vi "GSP_Manager_Slit.vi"() -> ()   [LabVIEW 2015]
uses:
  SystemUtil/ScriptArray.ctl
  SystemUtil/Script.ctl
  SystemUtil/MotorStates.ctl
  SystemUtil/ThreadStates.ctl
  Log/LogItem.ctl
  GSP_SLIT_Global.vi
  GUI/GSP_GUI_global.vi
  <vilib>/Utility/file.llb/Read From Spreadsheet File (DBL).vi
panel:
  in  "SLICER IN":bool
  in  "Slit":picture caption="Mask Is Out"
  in  "Mask bump":i32(slide) scale=-30.0..30.0
  in  "Hide Slit":bool
  in  "Slit Mask#":i32(ring) items=["<NO MASK>"]
  out "Last Error":errorcluster
  in  "CommandQ":string
  # "Mask"
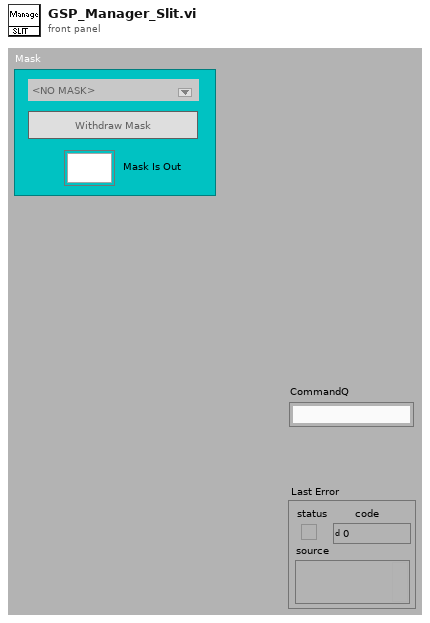
[diagram p1: front panel]
types:
  T1 = typedef "ScriptArray.ctl" = T2[]
  T2 = typedef "Script.ctl" = cluster{"Current Step":i32, "Commands":cluster{"Command":string, "Parameters":string}[]}
  T3 = cluster{"Trans Grab Mem Address":i32, "Trans Release Mem Address":i32, "Trans Home Mem Address":i32, "Trans Move Mem Address":i32, "Trans Open Mask Address":i32, "Trans Close Mask Address":i32, "Rot Home Mem Address":i32, "Rot Rotate Mem Address":i32}
  T4 = typedef "MotorStates.ctl" = enum16{"Ready", "Moving", "Uninitialized", "Error"}
  T5 = enum16{"POL (0)", "CPL (1)", "HLT (2)", "STP (3)", "RST (4)", "RVN (5)", "RPB (6)", "CLP (8)", "SDL (9)", "RUN (10)", "WRI (11)", "RRG (12)", "SPR (13)", "LPR (14)", "VMI (15)", "SSP (17)", "SSE (18)", "RIS (20)", "RIO (21)", "IMW (25)", "END (128)", "MAV (134)", "MRV (135)", "JRE (137)", "WCL (138)", "WCW (139)", "DLY (140)", "WDL (141)", "GCL (142)", "GOP (143)", "ZTG (144)", "ZTP (145)", "TTP (146)", "CME (147)", "CTC (148)", "TQL (149)", "AHC (150)", "ERL (151)", "OLP (152)", "WRP (154)", "IDT (155)", "LRP (156)", "VMP (159)", "RAV (160)", "RRV (161)", "JMP (162)", "JOI (162)", "CIS (163)", "CKS (164)", "CLC (165)", "KMC (167)", "MCT (168)", "FLC (169)", "EEM (170)", "DDB (171)", "DEM (171)", "PAC (172)", "ADL (173)", "BRT (174)", "MAT (176)", "MRT (177)", "RAT (178)", "RRT (179)", "SSD (180)", "KMR (181)", "KED (182)", "KDD (183)", "DIR (184)", "PRO (185)", "SIF (186)", "EDL (187)", "CIO (188)", "MDS (189)", "MDC (190)", "MDT (191)", "SEE (192)", "ARI (193)", "WBS (194)", "SCF (195)", "RSM (196)", "RLM (197)", "RSN (198)", "RLN (199)", "PCL (201)", "PCI (201)", "PRT (202)", "PRI (202)", "WBE (204)", "SOB (205)", "COB (206)", "ACR (207)", "PLR (208)", "CAI (211)", "LVT (212)", "OVT (213)", "MTT (214)", "CLC (215)", "PIM (216)", "VIM (217)", "TIM (218)", "AHM (219)", "SSL (221)", "TRU (222)", "RSD (223)", "EMT (225)", "DMT (226)", "EMD (227)", "DMD (228)", "HSM (229)", "AHD (230)", "PCM (231)", "PCG (232)", "XRV (233)", "XAV (234)", "XRT (235)", "XAT (236)", "GOC (237)", "JNA (238)", "JOR (239)", "PMC (240)", "PMV (241)", "PMX (242)", "DLC (243)", "SLC (244)", "PCP (245)", "ATR (248)", "PMO (249)", "JAN (250)", "EDH (251)", "DIF (252)", "IMS (253)", "IMQ (254)"}
  T6 = typedef "ThreadStates.ctl" = enum16{"Waiting", "Scripting", "Uninitialized", "Error"}
  T7 = cluster{"left":i16, "top":i16, "right":i16, "bottom":i16}
  T8 = cluster{"Width":u16, "Style":enum32{"Solid", "Dash", "Dot", "DashDot", "DashDotDot"}}
  T9 = enum16{"Launch", "Log", "Open", "Close", "Shutdown"}
  T10 = typedef "LogItem.ctl" = cluster{"error in (no error)":errorcluster, "Source":string, "Comment ":string}
  T11 = cluster{"left":i16, "bottom":i16, i16, "bottom":i16}
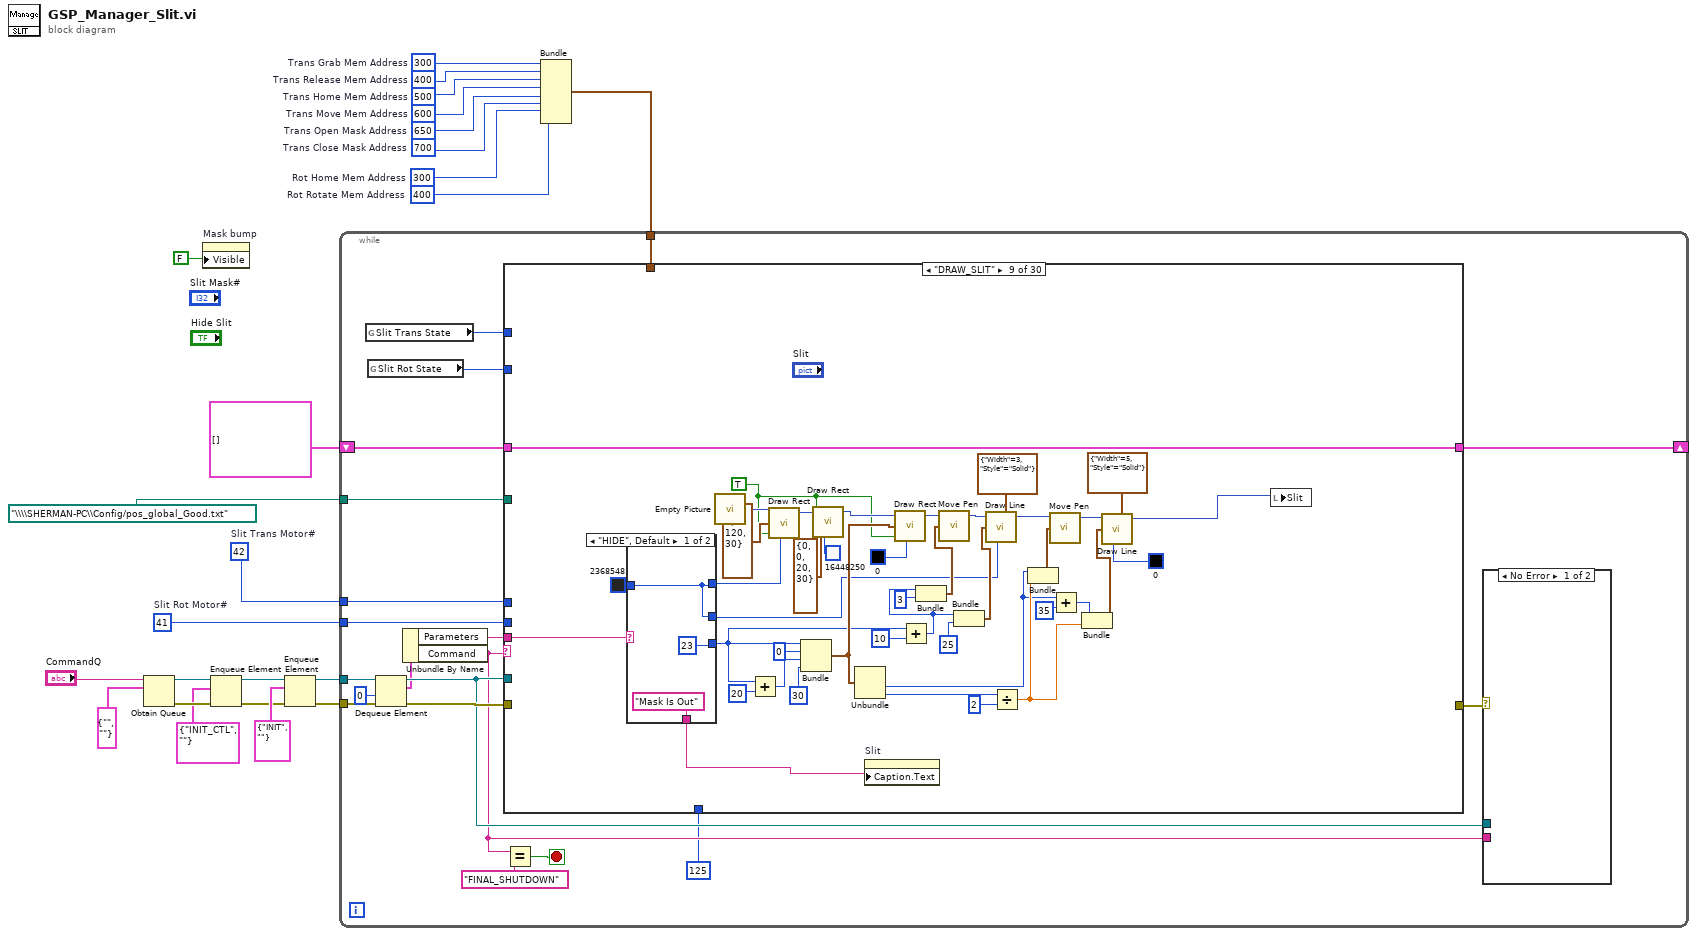
[diagram p0: block diagram]
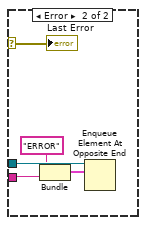
[diagram p2: hidden frame]
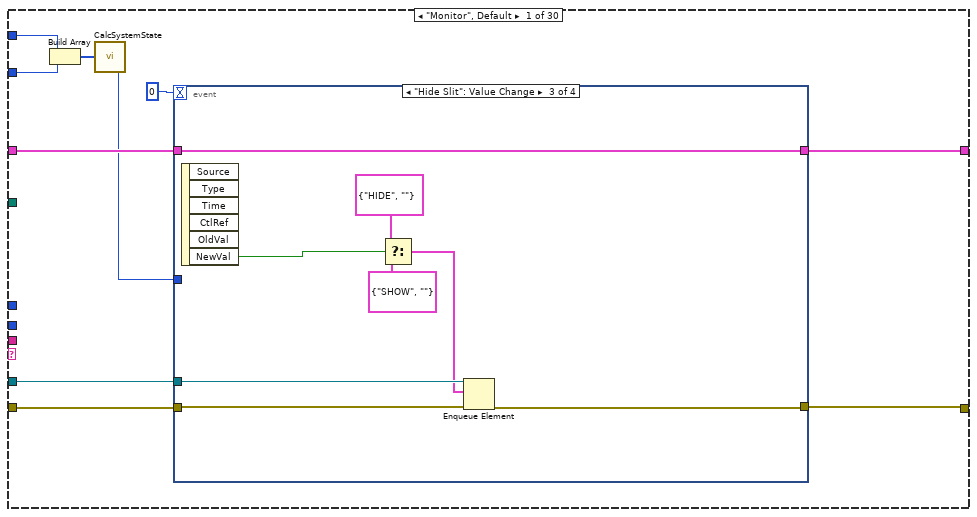
[diagram p3: hidden frame]
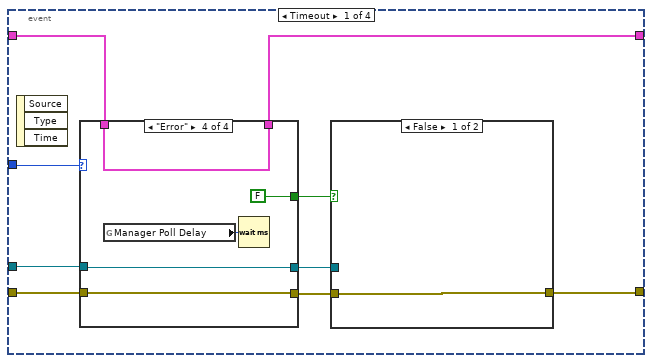
[diagram p4: hidden frame]
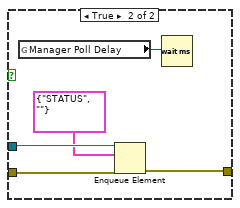
[diagram p5: hidden frame]
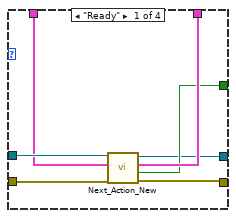
[diagram p6: hidden frame]
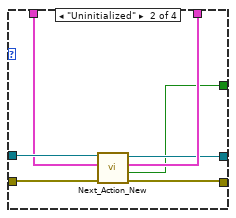
[diagram p7: hidden frame]
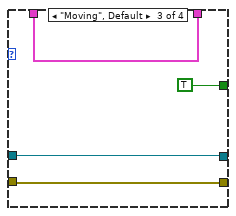
[diagram p8: hidden frame]
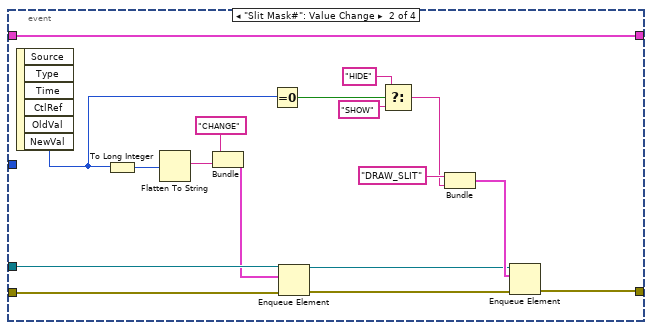
[diagram p9: hidden frame]
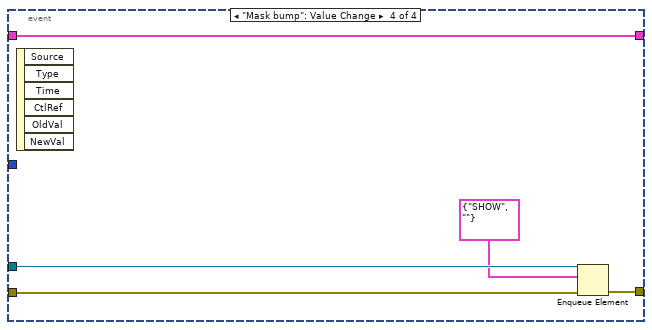
[diagram p10: hidden frame]
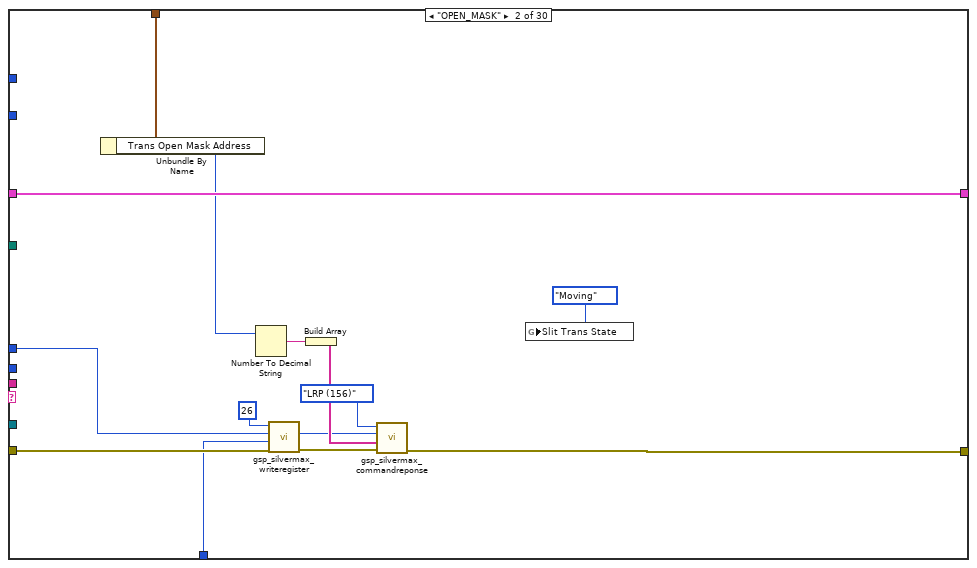
[diagram p11: hidden frame]
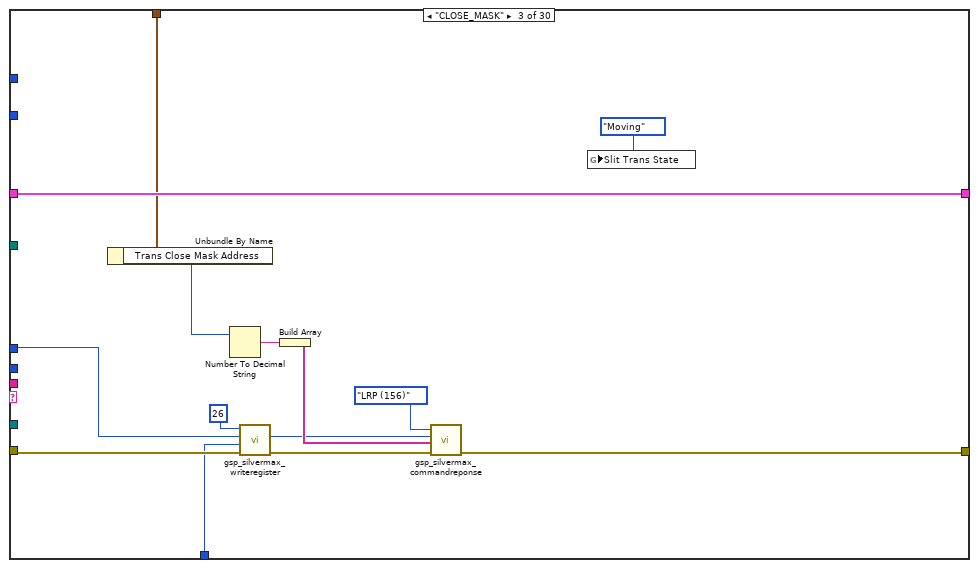
[diagram p12: hidden frame]
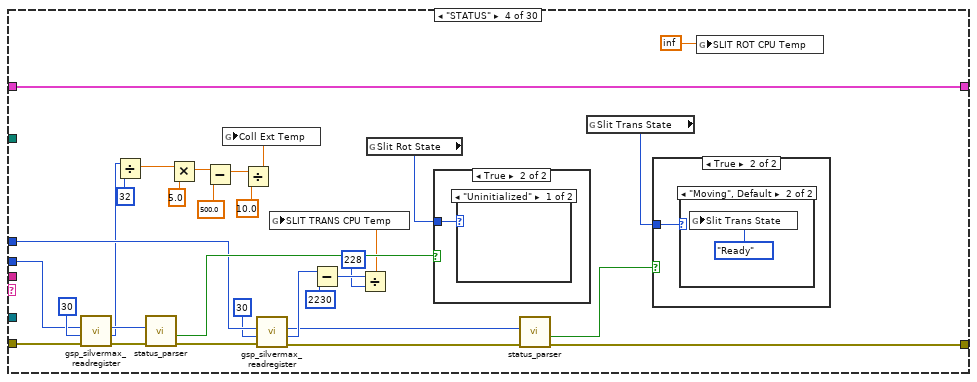
[diagram p13: hidden frame]
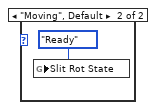
[diagram p17: hidden frame]
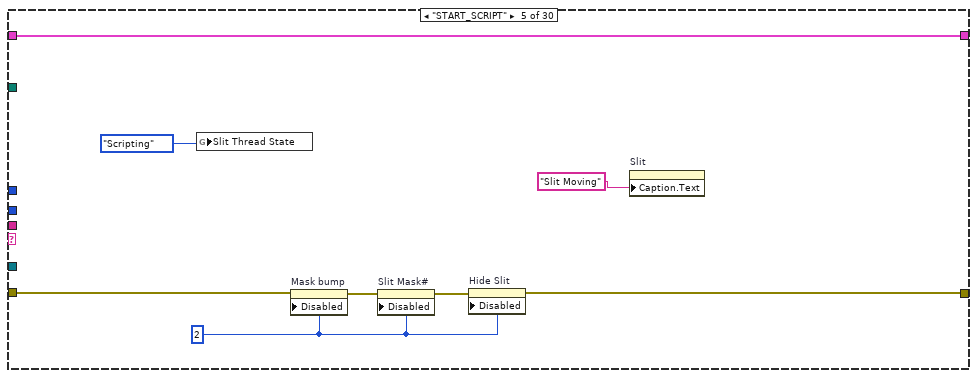
[diagram p18: hidden frame]
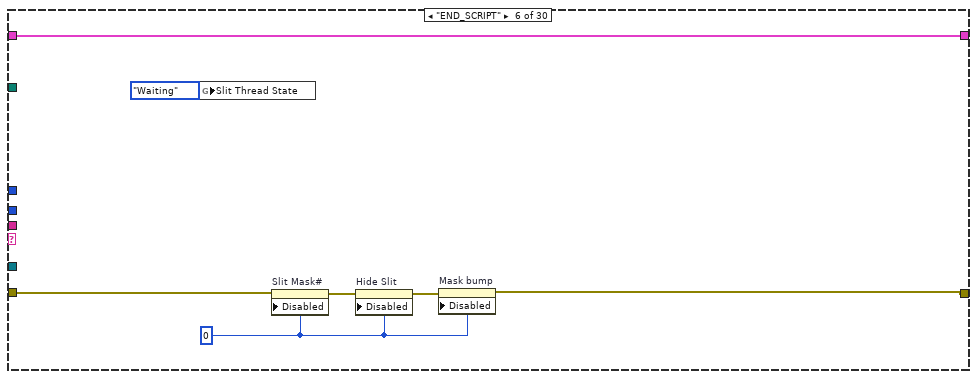
[diagram p19: hidden frame]
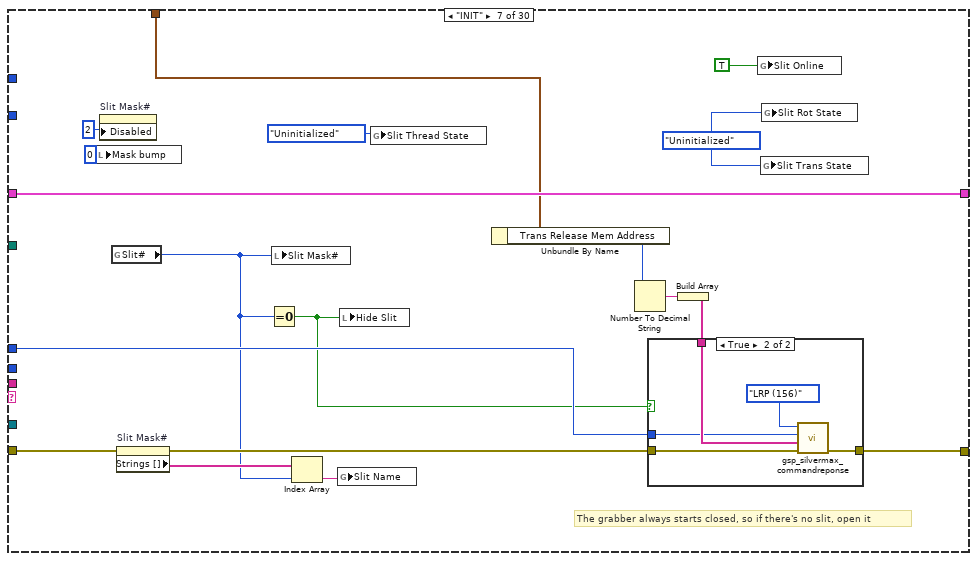
[diagram p20: hidden frame]
diagram:
  w16 = 300  # Trans Grab Mem Address
  w15 = 400  # Trans Release Mem Address
  w14 = 500  # Trans Home Mem Address
  w13 = 600  # Trans Move Mem Address
  w11 = 700  # Trans Close Mask Address
  w12 = 650  # Trans Open Mask Address
  w10 = 300  # Rot Home Mem Address
  w9 = 400  # Rot Rotate Mem Address
  w17 = u8 41  # Slit Rot Motor#
  w18 = u8 42  # Slit Trans Motor#
  n1 = Obtain Queue(name (unnamed)="CommandQ", element data type=cluster{"Command":string, "Parameters":string} {"Command"="", "Parameters"=""} ("Default Command")) -> (queue out=w4:refnum<queue>, error out=w5:errorcluster)  [unwired: 3 in, 1 out]
  n2 = property on="Mask bump" class="Slide (strict)"("Visible"=FALSE) -> ()  [unwired: 2 in, 2 out]
  n3 = Enqueue Element(queue=w4, element=cluster{"Command":string, "Parameters":string} {"Command"="INIT_CTL", "Parameters"=""}, error in (no error)=w5) -> (queue out=w7:refnum<queue>, error out=w6:errorcluster)  [unwired: 1 in, 1 out]
  n4 = Enqueue Element(queue=w7, element=cluster{"Command":string, "Parameters":string} {"Command"="INIT", "Parameters"=""}, error in (no error)=w6) -> (queue out=w24:refnum<queue>, error out=w23:errorcluster)  [unwired: 1 in, 1 out]
  n5 = Bundle("Trans Grab Mem Address"=w16, "Trans Release Mem Address"=w15, "Trans Home Mem Address"=w14, "Trans Move Mem Address"=w13, "Trans Open Mask Address"=w12, "Trans Close Mask Address"=w11, "Rot Home Mem Address"=w10, "Rot Rotate Mem Address"=w9) -> (w8:T3)  [unwired: 1 in]
  n6 = while {
    tunnel: w24 -> [w44]
    tunnel: w23 -> [w43]
    tunnel: w18 -> [w38]
    tunnel: w17 -> [w37]
    shift-right: [w36] -> _
    shift-left: T1 [] ("Operations") -> [w26]
    tunnel: w8 -> [w27]
    tunnel: path "\\\\SHERMAN-PC\\Config/pos_global_Good.txt" -> [w25]
    stop <- w33 stop-if-true
    n7 = global read "GSP_SLIT_Global.vi" "Slit Trans State"() -> (w28:T4)
    n8 = global read "GSP_SLIT_Global.vi" "Slit Rot State"() -> (w29:T4)
    n9 = Dequeue Element(queue=w44, timeout in ms (-1)=0, error in (no error)=w43) -> (queue out=w40:refnum<queue>, element=w35:cluster{"Command":string, "Parameters":string}, error out=w42:errorcluster)  [unwired: 1 out]
    n10 = Unbundle By Name(w35) -> ("Parameters"=w34:string, "Command"=w32:string)
    n11 = case shown="\"DRAW_SLIT\"" w32 {
      tunnel: w42 -> [w59 w136 w148 w182 w197 w204 w210 w239 _ w300 w310 w334 w363 w392 w397 w410 w424 w441 w459 w473 w492 w519 w545 w549 w568 w584 w626 w635 w638 _]
      tunnel: w40 -> [w50 _ _ _ _ _ _ _ _ w294 _ _ _ _ _ _ _ _ _ _ _ _ _ _ _ w590 w627 _ _ w664]
      tunnel: [w51 w128 w151 w167 w193 w201 w214 w239 _ w296 w309 w333 w365 w392 w397 w414 w419 w434 w463 w481 w494 w526 w545 w549 w577 w589 w622 w635 w650 _] -> w41
      tunnel: w38 -> [_ w135 w147 w170 _ _ w213 _ _ w298 _ _ _ _ _ w409 w423 w438 w458 w472 w493 w517 _ _ _ _ _ _ w642 _]
      tunnel: w37 -> [_ _ _ w181 _ _ _ _ _ w297 _ _ _ _ _ _ _ _ _ _ _ _ _ _ w581 _ _ _ w653 _]
      tunnel: w26 -> [w58 w141 w155 w184 w198 w205 w222 w240 w286 w301 w314 w338 w368 w396 w401 w404 w432 w439 w454 w470 w488 w522 w544 w548 w571 w592 w628 w637 w643 w658]
      tunnel: [w52 w141 w155 w184 w198 w205 w222 w240 w286 w301 w313 w337 w367 w395 w400 w404 w432 w439 w454 w470 w488 w522 w544 w548 w571 w591 w628 w636 w643 w657] -> w36
      tunnel: w34 -> [_ _ _ _ _ _ _ _ w247 _ w312 w336 w361 _ _ _ _ _ _ _ _ _ _ _ w566 _ _ _ _ _]
      tunnel: 125 ("Register Value") -> [_ w132 w145 _ _ _ _ _ _ _ _ _ _ _ _ _ _ _ _ _ _ _ _ _ _ _ _ _ _ _]
      tunnel: w29 -> [w55 _ _ _ _ _ _ _ _ _ w308 w332 _ _ _ _ _ _ _ _ _ _ _ _ _ w587 _ _ _ _]
      tunnel: w28 -> [w56 _ _ _ _ _ _ _ _ _ w307 w331 _ _ _ _ _ _ _ _ _ _ _ _ _ w588 _ _ _ _]
      tunnel: w27 -> [_ w131 w144 _ _ _ w215 _ _ _ _ _ _ _ _ w403 w422 w440 w453 w469 w487 w521 _ _ w565 _ _ _ w641 _]
      tunnel: w25 -> [_ _ _ _ _ _ _ w235 _ _ _ _ _ _ _ _ _ _ _ _ w485 w516 _ _ w555 _ _ _ _ _]
      frame "Monitor", Default {
        n12 = Build Array(w56, w55) -> (w57:T4[])
        n13 = call "CalcSystemState.vi"("Motor States"=w57) -> ("system state"=w53:T4)
        n14 = event shown="[2] \"Hide Slit\": Value Change" {
          selector: _ -> [_ _ _ _]
          dyn-events: _ -> [_ _ _ _]
          timeout: 0 -> [_ _ _ _]
          tunnel: w59 -> [w63 w113 w122 w126]
          tunnel: w58 -> [w65 w112 w120 w123]
          tunnel: w53 -> [w60 _ _ _]
          tunnel: [w61 w100 w115 w127] -> w51
          tunnel: [w64 w112 w120 w123] -> w52
          tunnel: w50 -> [w62 w114 w121 w125]
          event Timeout {
            n15 = event-data() -> ()  [unwired: 1 in, 3 out]
            n16 = case shown="\"Error\"" w60 {
              tunnel: [w81 w88 w90 w95] -> w68
              tunnel: [w80 w87 w89 w93] -> w64
              tunnel: [w79 w85 TRUE FALSE] -> w67
              tunnel: [w78 w86 w91 w94] -> w66
              tunnel: w63 -> [w77 w83 w90 w95]
              tunnel: w62 -> [w76 w84 w91 w94]
              tunnel: w65 -> [w75 w82 w89 w93]
              frame "Ready" {
                n17 = call "Next_Action_New.vi"("error in (no error)"=w77, "Operations"=w75, "queue in"=w76) -> ("error out"=w81:errorcluster, "No command?"=w79:bool, "Operations Out"=w80:T1, "queue out"=w78:refnum<queue>)  [unwired: 1 in]
              }
              frame "Uninitialized" {
                n18 = call "Next_Action_New.vi"("error in (no error)"=w83, "Operations"=w82, "queue in"=w84) -> ("error out"=w88:errorcluster, "No command?"=w85:bool, "Operations Out"=w87:T1, "queue out"=w86:refnum<queue>)  [unwired: 1 in]
              }
              frame "Moving", Default {
              }
              frame "Error" {
                n19 = global read "GSP_GUI_global.vi" "Manager Poll Delay"() -> (w97:u32)
                n20 = Wait (ms)(milliseconds to wait=w97) -> ()  [unwired: 1 out]
              }
            }
            n21 = case shown="False" w67 {
              tunnel: w68 -> [w69 w74]
              tunnel: w66 -> [_ w73]
              tunnel: [w69 w71] -> w61
              frame False {
              }
              frame True {
                n22 = global read "GSP_GUI_global.vi" "Manager Poll Delay"() -> (w72:u32)
                n23 = Enqueue Element(queue=w73, element=cluster{"Command":string, "Parameters":string} {"Command"="STATUS", "Parameters"=""}, error in (no error)=w74) -> (error out=w71:errorcluster)  [unwired: 1 in, 2 out]
                n24 = Wait (ms)(milliseconds to wait=w72) -> ()  [unwired: 1 out]
              }
            }
          }
          event "Slit Mask#": Value Change {
            n25 = event-data() -> ("NewVal"=w99:i32)  [unwired: 1 in, 5 out]
            n26 = To Long Integer(number=w99) -> (32bit integer=w111:i32)
            n27 = Flatten To String(anything=w111) -> (data string=w110:string)  [unwired: 3 in, 2 out]
            n28 = Bundle("CHANGE", "data string"=w110) -> (w108:cluster{string, "data string":string})  [unwired: 1 in]
            n29 = Equal To 0?(x=w99) -> (x = 0?=w98:bool)
            n30 = Enqueue Element(queue=w114, element=w108, error in (no error)=w113) -> (queue out=w102:refnum<queue>, error out=w101:errorcluster)  [unwired: 1 in, 1 out]
            n31 = Select(t="HIDE" ("Parameters"), s=w98, f="SHOW" ("Parameters")) -> (s? t:f=w104:string)
            n32 = Bundle("Command"="DRAW_SLIT", "Parameters"=w104) -> (w103:cluster{"Command":string, "Parameters":string})  [unwired: 1 in]
            n33 = Enqueue Element(queue=w102, element=w103, error in (no error)=w101) -> (error out=w100:errorcluster)  [unwired: 1 in, 2 out]
          }
          event "Hide Slit": Value Change {
            n34 = event-data() -> ("NewVal"=w116:bool)  [unwired: 1 in, 5 out]
            n35 = Select(t=cluster{"Command":string, "Parameters":string} {"Command"="HIDE", "Parameters"=""} ("element"), s=w116, f=cluster{"Command":string, "Parameters":string} {"Command"="SHOW", "Parameters"=""} ("element")) -> (s? t:f=w117:cluster{"Command":string, "Parameters":string})
            n36 = Enqueue Element(queue=w121, element=w117, error in (no error)=w122) -> (error out=w115:errorcluster)  [unwired: 1 in, 2 out]
          }
          event "Mask bump": Value Change {
            n37 = event-data() -> ()  [unwired: 1 in, 6 out]
            n38 = Enqueue Element(queue=w125, element=cluster{"Command":string, "Parameters":string} {"Command"="SHOW", "Parameters"=""}, error in (no error)=w126) -> (error out=w127:errorcluster)  [unwired: 1 in, 2 out]
          }
        }
      }
      frame "OPEN_MASK" {
        n39 = Unbundle By Name(w131) -> ("Trans Open Mask Address"=w130:i32)
        n40 = Number To Decimal String(number=w130) -> (decimal integer string=w139:string)  [unwired: 1 in]
        n41 = call "gsp_silvermax_writeregister.vi"("error in (no error)"=w136, "Register Value"=w132, "Motor #"=w135, "Register# (0)"=u8 26) -> ("error out"=w137:errorcluster, "Motor # dup"=w133:u8)  [unwired: 2 in]
        n42 = Build Array(w139) -> (w138:string[])
        n43 = call "gsp_silvermax_commandreponse.vi"("error in (no error)"=w137, "Parameters (none)"=w138, "Motor #"=w133, "Command"=T5."LRP (156)") -> ("error out"=w128:errorcluster)  [unwired: 3 out]
        n44 = global write "GSP_SLIT_Global.vi" "Slit Trans State"(MotorStates."Moving" ("Translation Mode")) -> ()
      }
      frame "CLOSE_MASK" {
        n45 = Unbundle By Name(w144) -> ("Trans Close Mask Address"=w143:i32)
        n46 = Number To Decimal String(number=w143) -> (decimal integer string=w153:string)  [unwired: 1 in]
        n47 = call "gsp_silvermax_writeregister.vi"("error in (no error)"=w148, "Register Value"=w145, "Motor #"=w147, "Register# (0)"=u8 26) -> ("error out"=w149:errorcluster, "Motor # dup"=w146:u8)  [unwired: 2 in]
        n48 = Build Array(w153) -> (w152:string[])
        n49 = call "gsp_silvermax_commandreponse.vi"("error in (no error)"=w149, "Parameters (none)"=w152, "Motor #"=w146, "Command"=T5."LRP (156)") -> ("error out"=w151:errorcluster)  [unwired: 3 out]
        n50 = global write "GSP_SLIT_Global.vi" "Slit Trans State"(MotorStates."Moving" ("Translation Mode")) -> ()
      }
      frame "STATUS" {
        n51 = call "gsp_silvermax_readregister.vi"("error in (no error)"=w182, "Register# (0)"=u8 30, "Motor #"=w181) -> ("error out"=w179:errorcluster, "Register Value"=w159:i32, "Motor # dup"=w180:u8)  [unwired: 2 in, 2 out]
        n52 = Divide(x=w159, y=32) -> (x/y=w166:dbl)
        n53 = call "status_parser.vi"("error in (no error)"=w179, "Motor #"=w180) -> ("error out"=w174:errorcluster, "Program Complete?"=w186:bool)  [unwired: 3 in, 1 out]
        n54 = Multiply(x=w166, y=5.0) -> (x*y=w164:dbl)
        n55 = Subtract(x=w164, y=500.0) -> (x-y=w162:dbl)
        n56 = Divide(x=w162, y=10.0) -> (x/y=w158:dbl)
        n57 = global write "GSP_SLIT_Global.vi" "Coll Ext Temp"(w158) -> ()
        n58 = call "gsp_silvermax_readregister.vi"("error in (no error)"=w174, "Register# (0)"=u8 30, "Motor #"=w170) -> ("error out"=w173:errorcluster, "Register Value"=w177:i32, "Motor # dup"=w172:u8)  [unwired: 2 in, 2 out]
        n59 = Subtract(x=w177, y=2230) -> (x-y=w176:i32)
        n60 = Divide(x=w176, y=228) -> (x/y=w171:dbl)
        n61 = global write "GSP_SLIT_Global.vi" "SLIT TRANS CPU Temp"(w171) -> ()
        n62 = global read "GSP_SLIT_Global.vi" "Slit Rot State"() -> (w157:T4)
        n63 = case shown="True" w186 {
          tunnel: w157 -> [_ w189]
          frame False {
          }
          frame True {
            n64 = case shown="\"Uninitialized\"" w189 {
              frame "Uninitialized" {
              }
              frame "Moving", Default {
                n65 = global write "GSP_SLIT_Global.vi" "Slit Rot State"(MotorStates."Ready" ("Rotation Mode")) -> ()
              }
            }
          }
        }
        n66 = call "status_parser.vi"("error in (no error)"=w173, "Motor #"=w172) -> ("error out"=w167:errorcluster, "Program Complete?"=w185:bool)  [unwired: 3 in, 1 out]
        n67 = global read "GSP_SLIT_Global.vi" "Slit Trans State"() -> (w156:T4)
        n68 = case shown="True" w185 {
          tunnel: w156 -> [_ w187]
          frame False {
          }
          frame True {
            n69 = case shown="\"Moving\", Default" w187 {
              frame "Uninitialized" {
              }
              frame "Moving", Default {
                n70 = global write "GSP_SLIT_Global.vi" "Slit Trans State"(MotorStates."Ready" ("Translation Mode")) -> ()
              }
            }
          }
        }
        n71 = global write "GSP_SLIT_Global.vi" "SLIT ROT CPU Temp"(inf) -> ()
      }
      frame "START_SCRIPT" {
        w194 = u8 2 ("Disabled")
        n72 = global write "GSP_SLIT_Global.vi" "Slit Thread State"(ThreadStates."Scripting" ("Thread state")) -> ()
        n73 = property on="Mask bump" class="Slide (strict)"(error in=w197, "Disabled"=w194) -> (error out=w196:errorcluster)  [unwired: 1 in, 1 out]
        n74 = property on="Slit Mask#" class="Ring (strict)"(error in=w196, "Disabled"=w194) -> (error out=w195:errorcluster)  [unwired: 1 in, 1 out]
        n75 = property on="Hide Slit" class="Bool (strict)"(error in=w195, "Disabled"=w194) -> (error out=w193:errorcluster)  [unwired: 1 in, 1 out]
        n76 = property on="Slit" class="Pict"("Caption.Text"="Slit Moving") -> ()  [unwired: 2 in, 2 out]
      }
      frame "END_SCRIPT" {
        w200 = u8 0 ("Disabled")
        n77 = global write "GSP_SLIT_Global.vi" "Slit Thread State"(ThreadStates."Waiting" ("Slit Thread State")) -> ()
        n78 = property on="Slit Mask#" class="Ring (strict)"(error in=w204, "Disabled"=w200) -> (error out=w203:errorcluster)  [unwired: 1 in, 1 out]
        n79 = property on="Hide Slit" class="Bool (strict)"(error in=w203, "Disabled"=w200) -> (error out=w202:errorcluster)  [unwired: 1 in, 1 out]
        n80 = property on="Mask bump" class="Slide (strict)"(error in=w202, "Disabled"=w200) -> (error out=w201:errorcluster)  [unwired: 1 in, 1 out]
      }
      frame "INIT" {
        w221 = MotorStates."Uninitialized" ("Rotation Mode")
        # "The grabber always starts closed, so if there's no slit, open it"
        n81 = local write "Mask bump"(0 ("Mask bump")) -> ()
        n82 = property on="Slit Mask#" class="Ring (strict)"("Disabled"=u8 2) -> ()  [unwired: 2 in, 2 out]
        n83 = global read "GSP_SLIT_Global.vi" "Slit#"() -> (w207:i32)
        n84 = property on="Slit Mask#" class="Ring (strict)"(error in=w210) -> (error out=w208:errorcluster, "Strings []"=w209:string[])  [unwired: 1 in, 1 out]
        n85 = Equal To 0?(x=w207) -> (x = 0?=w212:bool)
        n86 = local write "Slit Mask#"(w207) -> ()
        n87 = Index Array(array=w209, index=w207) -> (element=w206:string)
        n88 = global write "GSP_SLIT_Global.vi" "Slit Name"(w206) -> ()
        n89 = local write "Hide Slit"(w212) -> ()
        n90 = global write "GSP_SLIT_Global.vi" "Slit Thread State"(ThreadStates."Uninitialized" ("Thread state")) -> ()
        n91 = Unbundle By Name(w215) -> ("Trans Release Mem Address"=w216:i32)
        n92 = Number To Decimal String(number=w216) -> (decimal integer string=w218:string)  [unwired: 1 in]
        n93 = Build Array(w218) -> (w217:string[])
        n94 = case shown="True" w212 {
          tunnel: w217 -> [_ w228]
          tunnel: w208 -> [w224 w227]
          tunnel: [w224 w226] -> w214
          tunnel: w213 -> [_ w225]
          frame False {
          }
          frame True {
            n95 = call "gsp_silvermax_commandreponse.vi"("error in (no error)"=w227, "Parameters (none)"=w228, "Motor #"=w225, "Command"=T5."LRP (156)") -> ("error out"=w226:errorcluster)  [unwired: 3 out]
          }
        }
        n96 = global write "GSP_SLIT_Global.vi" "Slit Online"(TRUE ("CS Online")) -> ()
        n97 = global write "GSP_SLIT_Global.vi" "Slit Trans State"(w221) -> ()
        n98 = global write "GSP_SLIT_Global.vi" "Slit Rot State"(w221) -> ()
      }
      frame "INIT_CTL" {
        w233 = 0 ("disabled index (col)")
        n99 = call-poly <vilib>:"Read From Spreadsheet File.vi"("number of rows (all:-1)"=2, "file path (dialog if empty)"=w235) -> ("all rows"=w234:dbl[][])  [unwired: 5 in, 4 out]
        n100 = Index Array(array=w234, index (row)=0 ("index"), index (col)=w233) -> (element=w231:dbl)
        n101 = Index Array(array=w234, index (row)=1 ("index"), index (col)=w233) -> (element=w232:dbl)
        n102 = global read "GSP_GUI_global.vi" "Slit Mask Names"() -> (w244:string[])
        n103 = global write "GSP_SLIT_Global.vi" "Carousel Pos"(w232) -> ()
        n104 = global write "GSP_SLIT_Global.vi" "Slit#"(w231) -> ()
        n105 = Insert Into Array(array=w244, index=0, new element="<NO MASK>" ("new element/subarray")) -> (w241:string[])
        n106 = property on="Slit Mask#" class="Ring (strict)"("Strings []"=w241) -> ()  [unwired: 2 in, 2 out]
        n107 = property on="SLICER IN" class="Bool"("Visible"=FALSE) -> ()  [unwired: 2 in, 2 out]
      }
      frame "DRAW_SLIT" {
        w250 = TRUE ("fill?(F)")
        n108 = case shown="\"HIDE\", Default" w247 {
          tunnel: [i16 23 ("left") i16 0 ("left")] -> w260
          tunnel: [w288 w291] -> w255
          tunnel: [w288 u32 16448250 ("color(black)")] -> w254
          tunnel: u32 2368548 ("color(black)") -> [w288 w291]
          tunnel: ["Mask Is Out" ("Caption.Text") "Mask Is In" ("Caption.Text")] -> w245
          frame "HIDE", Default {
          }
          frame "SHOW" {
          }
        }
        n109 = call "Empty Picture"() -> ("empty picture"=w257:picture)
        n110 = Add(x=w260, y=i16 20 ("right")) -> (x+y=w262:i16)
        n111 = call <vilib>:"Draw Rect.vi"("picture"=w257, "rect"=T7 {"left"=0, "top"=0, "right"=120, "bottom"=30}, "fill?(F)"=w250, "color(black)"=w255) -> ("new picture"=w252:picture)  [unwired: 5 in]
        n112 = Bundle("left"=w260, "bottom"=i16 0, w262, "bottom"=i16 30) -> (w265:T11)  [unwired: 1 in]
        n113 = call <vilib>:"Draw Rect.vi"("picture"=w252, "rect"=T7 {"left"=0, "top"=0, "right"=20, "bottom"=30}, "fill?(F)"=w250, "color(black)"=u32 16448250) -> ("new picture"=w251:picture)  [unwired: 5 in]
        n114 = Unbundle(w265) -> (w266:i16, "bottom"=w272:i16)  [unwired: 2 out]
        n115 = property on="Slit" class="Pict"("Caption.Text"=w245) -> ()  [unwired: 2 in, 2 out]
        n116 = call <vilib>:"Draw Rect.vi"("picture"=w251, "rect"=w265, "fill?(F)"=w250, "color(black)"=u32 0) -> ("new picture"=w284:picture)  [unwired: 5 in]
        n117 = Add(x=w260, y=i16 10) -> (x+y=w259:i16)
        n118 = Bundle(w259, "y"=i16 3) -> (w277:cluster{i16, "y":i16})  [unwired: 1 in]
        n119 = call <vilib>:"Move Pen.vi"("new position"=w277, "picture"=w284) -> ("new picture"=w283:picture)  [unwired: 3 in]
        n120 = Bundle(w259, "y"=i16 25) -> (w275:cluster{i16, "y":i16})  [unwired: 1 in]
        n121 = call <vilib>:"Draw Line.vi"("picture"=w283, "end point"=w275, "color(black)"=w254, "pen"=T8 {"Width"=3, "Style"=enum."Solid"}) -> ("new picture"=w281:picture)  [unwired: 5 in]
        n122 = Divide(x=w272, y=i16 2) -> (x/y=w269:dbl)
        n123 = Bundle(w266, w269) -> (w273:cluster{i16, dbl})  [unwired: 1 in]
        n124 = call <vilib>:"Move Pen.vi"("new position"=w273, "picture"=w281) -> ("new picture"=w280:picture)  [unwired: 3 in]
        n125 = Add(x=w266, y=i8 35) -> (x+y=w268:i16)
        n126 = Bundle(w268, w269) -> (w270:cluster{i16, dbl})  [unwired: 1 in]
        n127 = call <vilib>:"Draw Line.vi"("picture"=w280, "end point"=w270, "color(black)"=u32 0, "pen"=T8 {"Width"=5, "Style"=enum."Solid"}) -> ("new picture"=w246:picture)  [unwired: 5 in]
        n128 = local write "Slit"(w246) -> ()
      }
      frame "RESTART" {
        n129 = call "Silvermax_restart.vi"("error in (no error)"=w300, "Motor #"=w298) -> ("error out"=w299:errorcluster)  [unwired: 4 in, 1 out]
        n130 = call "Silvermax_restart.vi"("error in (no error)"=w299, "Motor #"=w297) -> ("error out"=w295:errorcluster)  [unwired: 4 in, 1 out]
        n131 = case shown="No Error" w295 {
          selector: w295 -> [w304 w306]
          tunnel: [w303 w306] -> w296
          tunnel: w294 -> [w305 _]
          frame No Error {
            n132 = Enqueue Element(queue=w305, element=cluster{"Command":string, "Parameters":string} {"Command"="INIT", "Parameters"=""}, error in (no error)=w304) -> (error out=w303:errorcluster)  [unwired: 1 in, 2 out]
          }
          frame Error {
          }
        }
      }
      frame "CHANGE" {
        n133 = call "Slit_allow_move.vi"("Translation Mode"=w307, "Rotation Mode"=w308) -> ("Allow Move?"=w311:bool)
        n134 = case shown="True" w311 {
          tunnel: w314 -> [w322 w330]
          tunnel: [w322 w329] -> w313
          tunnel: w312 -> [_ w325]
          tunnel: w310 -> [w321 w328]
          tunnel: [w320 w328] -> w309
          frame False {
            n135 = Bundle By Name(cluster=T10 {"error in (no error)"={"status"=FALSE, "code"=0, "source"=""}, "Source"="", "Comment "=""} ("Log"), "Source"="Slit Manager", "Comment"="Cannot change slit") -> (w315:T10)
            n136 = call "GSP_Logger_Handler.vi"("error in (no error)"=w321, "Log"=w315, "Actions"=T9."Log") -> ("error out"=w320:errorcluster)  [unwired: 4 in]
          }
          frame True {
            n137 = Bundle("CHANGE_START", "Parameters"=w325) -> (w324:cluster{string, "Parameters":string})  [unwired: 1 in]
            n138 = Build Array(w324) -> (w323:cluster{string, "Parameters":string}[])
            n139 = call "Build_Script.vi"("Commands"=w323) -> ("script out"=w327:T2)  [unwired: 4 in]
            n140 = Insert Into Array(array=w330, new element=w327) -> (w329:T1)  [unwired: 1 in]
          }
        }
      }
      frame "ROTATE_ONLY" {
        n141 = call "Slit_allow_move.vi"("Translation Mode"=w331, "Rotation Mode"=w332) -> ("Allow Move?"=w335:bool)
        n142 = case shown="True" w335 {
          tunnel: w338 -> [w346 w359]
          tunnel: [w346 w358] -> w337
          tunnel: w336 -> [_ w353]
          tunnel: w334 -> [w345 w357]
          tunnel: [w344 w357] -> w333
          frame False {
            n143 = Bundle By Name(cluster=T10 {"error in (no error)"={"status"=FALSE, "code"=0, "source"=""}, "Source"="", "Comment "=""} ("Log"), "Source"="Slit Manager", "Comment"="Cannot change slit") -> (w339:T10)
            n144 = call "GSP_Logger_Handler.vi"("error in (no error)"=w345, "Log"=w339, "Actions"=T9."Log") -> ("error out"=w344:errorcluster)  [unwired: 4 in]
          }
          frame True {
            w351 = ""
            n145 = Bundle("String"="START_SCRIPT", w351) -> (w350:cluster{"String":string, string})  [unwired: 1 in]
            n146 = Bundle("String"="ROTATE", "Parameters"=w353) -> (w349:cluster{"String":string, "Parameters":string})  [unwired: 1 in]
            n147 = Bundle("String"="END_SCRIPT", w351) -> (w348:cluster{"String":string, string})  [unwired: 1 in]
            n148 = Build Array(w350, w349, w348) -> (w347:cluster{"String":string, "Parameters":string}[])
            n149 = call "Build_Script.vi"("Commands"=w347) -> ("script out"=w356:T2)  [unwired: 4 in]
            n150 = Insert Into Array(array=w359, new element=w356) -> (w358:T1)  [unwired: 1 in]
          }
        }
      }
      frame "CHANGE_START" {
        n151 = Unflatten From String(type=0, binary string=w361) -> (value=w362:i32)  [unwired: 3 in, 2 out]
        n152 = global read "GSP_SLIT_Global.vi" "Slit#"() -> (w360:i32)
        n153 = Equal?(x=w360, y=w362) -> (x = y?=w366:bool)
        n154 = case shown="False" w366 {
          tunnel: w368 -> [w379 w391]
          tunnel: [w369 w391] -> w367
          tunnel: [w374 w390] -> w365
          tunnel: w363 -> [w374 w390]
          tunnel: w362 -> [w376 _]
          tunnel: w361 -> [_ _]
          frame False {
            n155 = Equal?(x=w376, y=0) -> (x = y?=w372:bool)
            n156 = global read "GSP_SLIT_Global.vi" "Slit#"() -> (w373:i32)
            n157 = local write "Hide Slit"(w372) -> ()
            n158 = call "SLIT_generate_script.vi"("Script Type"=enum16{"Home", "Change"}."Change", "Current Slit#"=w373, "Slit#"=w376) -> ("script out"=w375:T2)
            n159 = Insert Into Array(array=w379, new element=w375) -> (w371:T1)  [unwired: 1 in]
            n160 = case shown="True" w372 {
              tunnel: [w380 w385] -> w370
              frame False {
                n161 = Bundle("Command"="DRAW_SLIT", "Parameters"="SHOW") -> (w382:cluster{"Command":string, "Parameters":string})  [unwired: 1 in]
                n162 = Build Array(w382) -> (w381:cluster{"Command":string, "Parameters":string}[])
                n163 = call "Build_Script.vi"("Commands"=w381) -> ("script out"=w380:T2)  [unwired: 4 in]
              }
              frame True {
                n164 = Bundle("Command"="DRAW_SLIT", "Parameters"="HIDE") -> (w387:cluster{"Command":string, "Parameters":string})  [unwired: 1 in]
                n165 = Build Array(w387) -> (w386:cluster{"Command":string, "Parameters":string}[])
                n166 = call "Build_Script.vi"("Commands"=w386) -> ("script out"=w385:T2)  [unwired: 4 in]
              }
            }
            n167 = Insert Into Array(array=w371, new element=w370) -> (w369:T1)  [unwired: 1 in]
          }
          frame True {
          }
        }
      }
      frame "HIDE" {
        n168 = call "Build_Script.vi"("Commands"=cluster{"Command":string, "Parameters":string}[] [{"Command"="START_SCRIPT", "Parameters"=""}, {"Command"="MOVE_HIDE_POS", "Parameters"=""}, {"Command"="END_SCRIPT", "Parameters"=""}, {"Command"="DRAW_SLIT", "Parameters"="HIDE"}]) -> ("script out"=w394:T2)  [unwired: 4 in]
        n169 = Insert Into Array(array=w396, new element=w394) -> (w395:T1)  [unwired: 1 in]
      }
      frame "SHOW" {
        n170 = call "Build_Script.vi"("Commands"=cluster{"Command":string, "Parameters":string}[] [{"Command"="START_SCRIPT", "Parameters"=""}, {"Command"="MOVE_DETENT_POS", "Parameters"=""}, {"Command"="END_SCRIPT", "Parameters"=""}, {"Command"="DRAW_SLIT", "Parameters"="SHOW"}, {"Command"="", "Parameters"=""}]) -> ("script out"=w398:T2)  [unwired: 4 in]
        n171 = Insert Into Array(array=w401, new element=w398) -> (w400:T1)  [unwired: 1 in]
      }
      frame "MOVE_LOAD_POS" {
        n172 = global read "GSP_SLIT_Global.vi" "Grab Position"() -> (w407:i32)
        n173 = Unbundle By Name(w403) -> ("Trans Move Mem Address"=w402:i32)
        n174 = Number To Decimal String(number=w402) -> (decimal integer string=w406:string)  [unwired: 1 in]
        n175 = call "gsp_silvermax_writeregister.vi"("error in (no error)"=w410, "Register Value"=w407, "Motor #"=w409, "Register# (0)"=u8 25) -> ("error out"=w411:errorcluster, "Motor # dup"=w412:u8)  [unwired: 2 in]
        n176 = Build Array(w406) -> (w405:string[])
        n177 = call "gsp_silvermax_commandreponse.vi"("error in (no error)"=w411, "Parameters (none)"=w405, "Motor #"=w412, "Command"=T5."LRP (156)") -> ("error out"=w415:errorcluster)  [unwired: 3 out]
        n178 = case shown="No Error" w415 {
          selector: w415 -> [w416 w418]
          tunnel: [w416 w418] -> w414
          frame No Error {
            n179 = global write "GSP_SLIT_Global.vi" "Slit Trans State"(MotorStates."Moving" ("Translation Mode")) -> ()
          }
          frame Error {
          }
        }
      }
      frame "MOVE_HIDE_POS" {
        n180 = global read "GSP_SLIT_Global.vi" "No Slit Position"() -> (w427:i32)
        n181 = Unbundle By Name(w422) -> ("Trans Move Mem Address"=w421:i32)
        n182 = Number To Decimal String(number=w421) -> (decimal integer string=w426:string)  [unwired: 1 in]
        n183 = call "gsp_silvermax_writeregister.vi"("error in (no error)"=w424, "Register Value"=w427, "Motor #"=w423, "Register# (0)"=u8 25) -> ("error out"=w429:errorcluster, "Motor # dup"=w430:u8)  [unwired: 2 in]
        n184 = Build Array(w426) -> (w425:string[])
        n185 = call "gsp_silvermax_commandreponse.vi"("error in (no error)"=w429, "Parameters (none)"=w425, "Motor #"=w430, "Command"=T5."LRP (156)") -> ("error out"=w419:errorcluster)  [unwired: 3 out]
        n186 = global write "GSP_SLIT_Global.vi" "Slit Trans State"(MotorStates."Moving" ("Translation Mode")) -> ()
      }
      frame "MOVE_DETENT_PLUS" {
        n187 = global read "GSP_SLIT_Global.vi" "Detent Position"() -> (w437:i32)
        n188 = Unbundle By Name(w440) -> ("Trans Move Mem Address"=w442:i32)
        n189 = Add(x=12000, y=w437) -> (x+y=w433:i32)
        n190 = Number To Decimal String(number=w442) -> (decimal integer string=w444:string)  [unwired: 1 in]
        n191 = Build Array(w444) -> (w443:string[])
        n192 = call "gsp_silvermax_writeregister.vi"("error in (no error)"=w441, "Register Value"=w433, "Motor #"=w438, "Register# (0)"=u8 25) -> ("error out"=w446:errorcluster, "Motor # dup"=w445:u8)  [unwired: 2 in]
        n193 = call "gsp_silvermax_commandreponse.vi"("error in (no error)"=w446, "Parameters (none)"=w443, "Motor #"=w445, "Command"=T5."LRP (156)") -> ("error out"=w434:errorcluster)  [unwired: 3 out]
        n194 = global write "GSP_SLIT_Global.vi" "Slit Trans State"(MotorStates."Moving" ("Translation Mode")) -> ()
      }
      frame "MOVE_DETENT_POS" {
        n195 = Unbundle By Name(w453) -> ("Trans Move Mem Address"=w452:i32)
        n196 = global read "GSP_SLIT_Global.vi" "Detent Position"() -> (w451:i32)
        n197 = Add(x="Mask bump", y=w451) -> (x+y=w450:i32)
        n198 = Number To Decimal String(number=w452) -> (decimal integer string=w456:string)  [unwired: 1 in]
        n199 = Build Array(w456) -> (w455:string[])
        n200 = call "gsp_silvermax_writeregister.vi"("error in (no error)"=w459, "Register Value"=w450, "Motor #"=w458, "Register# (0)"=u8 25) -> ("error out"=w460:errorcluster, "Motor # dup"=w457:u8)  [unwired: 2 in]
        n201 = call "gsp_silvermax_commandreponse.vi"("error in (no error)"=w460, "Parameters (none)"=w455, "Motor #"=w457, "Command"=T5."LRP (156)") -> ("error out"=w464:errorcluster)  [unwired: 3 out]
        n202 = case shown="No Error" w464 {
          selector: w464 -> [w465 w467]
          tunnel: [w465 w467] -> w463
          frame No Error {
            n203 = global write "GSP_SLIT_Global.vi" "Slit Trans State"(MotorStates."Moving" ("Translation Mode")) -> ()
          }
          frame Error {
          }
        }
      }
      frame "MOVE_CLEAR_POS" {
        n204 = Unbundle By Name(w469) -> ("Trans Move Mem Address"=w468:i32)
        n205 = global read "GSP_SLIT_Global.vi" "Clear Position"() -> (w478:i32)
        n206 = Number To Decimal String(number=w468) -> (decimal integer string=w475:string)  [unwired: 1 in]
        n207 = Build Array(w475) -> (w474:string[])
        n208 = call "gsp_silvermax_writeregister.vi"("error in (no error)"=w473, "Register Value"=w478, "Motor #"=w472, "Register# (0)"=u8 25) -> ("error out"=w477:errorcluster, "Motor # dup"=w476:u8)  [unwired: 2 in]
        n209 = call "gsp_silvermax_commandreponse.vi"("error in (no error)"=w477, "Parameters (none)"=w474, "Motor #"=w476, "Command"=T5."LRP (156)") -> ("error out"=w471:errorcluster)  [unwired: 3 out]
        n210 = case shown="No Error" w471 {
          selector: w471 -> [w482 w484]
          tunnel: [w482 w484] -> w481
          frame No Error {
            n211 = global write "GSP_SLIT_Global.vi" "Slit Trans State"(MotorStates."Moving" ("Translation Mode")) -> ()
          }
          frame Error {
          }
        }
      }
      frame "RELEASE" {
        n212 = Unbundle By Name(w487) -> ("Trans Release Mem Address"=w486:i32)
        n213 = Number To Decimal String(number=w486) -> (decimal integer string=w490:string)  [unwired: 1 in]
        n214 = Build Array(w490) -> (w489:string[])
        n215 = call "gsp_silvermax_commandreponse.vi"("error in (no error)"=w492, "Parameters (none)"=w489, "Motor #"=w493, "Command"=T5."LRP (156)") -> ("error out"=w495:errorcluster)  [unwired: 3 out]
        n216 = case shown="No Error" w495 {
          selector: w495 -> [w511 w515]
          tunnel: [w508 w515] -> w494
          tunnel: w485 -> [w499 _]
          frame No Error {
            w512 = 0 ("Current Slit#")
            n217 = global read "GSP_SLIT_Global.vi" "Carousel Pos"() -> (w501:i32)
            n218 = Delete(path (use dialog)=w499) -> (deleted path=w500:path)  [unwired: 4 in, 2 out]
            n219 = property on="Slit Mask#" class="Ring (strict)"(error in=w511) -> (error out=w508:errorcluster, "Strings []"=w510:string[])  [unwired: 1 in, 1 out]
            n220 = Number To Decimal String(number=0) -> (decimal integer string=w506:string)  [unwired: 1 in]
            n221 = Number To Decimal String(number=w501) -> (decimal integer string=w496:string)  [unwired: 1 in]
            n222 = Concatenate Strings("\r\n", w496) -> (w498:string)
            n223 = call <vilib>:"Write Characters To File.vi"("append to file? (new file:F)"=FALSE, "character string"=w506, "file path (dialog if empty)"=w500) -> ("new file path (Not A Path if cancelled)"=w502:path)  [unwired: 2 in]
            n224 = call <vilib>:"Write Characters To File.vi"("append to file? (new file:F)"=TRUE, "character string"=w498, "file path (dialog if empty)"=w502) -> ()  [unwired: 2 in, 1 out]
            n225 = Index Array(array=w510, index=0) -> (element=w507:string)
            n226 = global write "GSP_SLIT_Global.vi" "Slit Name"(w507) -> ()
            n227 = global write "GSP_SLIT_Global.vi" "Slit Trans State"(MotorStates."Moving" ("Translation Mode")) -> ()
            n228 = Wait (ms)(milliseconds to wait=u32 500) -> ()  [unwired: 1 out]
            n229 = local write "Slit Mask#"(w512) -> ()
            n230 = global write "GSP_SLIT_Global.vi" "Slit#"(w512) -> ()
          }
          frame Error {
          }
        }
      }
      frame "GRAB" {
        n231 = Unbundle By Name(w521) -> ("Trans Grab Mem Address"=w520:i32)
        n232 = Number To Decimal String(number=w520) -> (decimal integer string=w524:string)  [unwired: 1 in]
        n233 = Build Array(w524) -> (w523:string[])
        n234 = call "gsp_silvermax_commandreponse.vi"("error in (no error)"=w519, "Parameters (none)"=w523, "Motor #"=w517, "Command"=T5."LRP (156)") -> ("error out"=w527:errorcluster)  [unwired: 3 out]
        n235 = case shown="No Error" w527 {
          selector: w527 -> [w540 w542]
          tunnel: [w538 w542] -> w526
          tunnel: w516 -> [w532 _]
          frame No Error {
            n236 = global read "GSP_SLIT_Global.vi" "Carousel Pos"() -> (w536:i32)
            n237 = property on="Slit Mask#" class="Ring (strict)"(error in=w540) -> (error out=w538:errorcluster, "Strings []"=w539:string[])  [unwired: 1 in, 1 out]
            n238 = Delete(path (use dialog)=w532) -> (deleted path=w531:path)  [unwired: 4 in, 2 out]
            n239 = global write "GSP_SLIT_Global.vi" "Slit#"(w536) -> ()
            n240 = Index Array(array=w539, index=w536) -> (element=w537:string)
            n241 = local write "Slit Mask#"(w536) -> ()
            n242 = global write "GSP_SLIT_Global.vi" "Slit Name"(w537) -> ()
            n243 = Number To Decimal String(number=w536) -> (decimal integer string=w528:string)  [unwired: 1 in]
            n244 = call <vilib>:"Write Characters To File.vi"("append to file? (new file:F)"=FALSE, "character string"=w528, "file path (dialog if empty)"=w531) -> ("new file path (Not A Path if cancelled)"=w533:path)  [unwired: 2 in]
            n245 = Concatenate Strings("\r\n", w528) -> (w530:string)
            n246 = Wait (ms)(milliseconds to wait=u32 500) -> ()  [unwired: 1 out]
            n247 = call <vilib>:"Write Characters To File.vi"("append to file? (new file:F)"=TRUE, "character string"=w530, "file path (dialog if empty)"=w533) -> ()  [unwired: 2 in, 1 out]
          }
          frame Error {
          }
        }
        n248 = global write "GSP_SLIT_Global.vi" "Slit Trans State"(MotorStates."Moving" ("Translation Mode")) -> ()
      }
      frame "DISABLE_SELECTION" {
        n249 = property on="Slit Mask#" class="Ring (strict)"("Disabled"=u8 2) -> ()  [unwired: 2 in, 2 out]
        n250 = property on="SLICER IN" class="Bool"("Visible"=TRUE) -> ()  [unwired: 2 in, 2 out]
      }
      frame "ENABLE_SELECTION" {
        n251 = property on="Slit Mask#" class="Ring (strict)"("Disabled"=u8 0) -> ()  [unwired: 2 in, 2 out]
        n252 = property on="SLICER IN" class="Bool"("Visible"=FALSE) -> ()  [unwired: 2 in, 2 out]
      }
      frame "ROTATE" {
        n253 = Unbundle By Name(w565) -> ("Rot Rotate Mem Address"=w564:i32)
        n254 = Unflatten From String(type=0, binary string=w566) -> (value=w563:i32)  [unwired: 3 in, 2 out]
        n255 = To Unsigned Word Integer(number=w563) -> (unsigned 16bit integer=w556:u16)
        n256 = global read "GSP_SLIT_Global.vi" "Counts per Position"() -> (w575:dbl)
        n257 = To Double Precision Float(number=w563) -> (double precision float=w583:dbl)
        n258 = global read "GSP_SLIT_Global.vi" "Offset to first Position"() -> (w572:i32)
        n259 = global write "GSP_SLIT_Global.vi" "Carousel Pos"(w556) -> ()
        n260 = Multiply(x=w583, y=w575) -> (x*y=w582:dbl)
        n261 = To Long Integer(number=w582) -> (32bit integer=w576:i32)
        n262 = Number To Decimal String(number=w564) -> (decimal integer string=w574:string)  [unwired: 1 in]
        n263 = Add(x=w576, y=w572) -> (x+y=w570:i32)
        n264 = Build Array(w574) -> (w573:string[])
        n265 = call "gsp_silvermax_writeregister.vi"("error in (no error)"=w568, "Register Value"=w570, "Motor #"=w581, "Register# (0)"=u8 25) -> ("error out"=w579:errorcluster, "Motor # dup"=w578:u8)  [unwired: 2 in]
        n266 = Delete(path (use dialog)=w555) -> (deleted path=w554:path)  [unwired: 4 in, 2 out]
        n267 = call "gsp_silvermax_commandreponse.vi"("error in (no error)"=w579, "Parameters (none)"=w573, "Motor #"=w578, "Command"=T5."LRP (156)") -> ("error out"=w577:errorcluster)  [unwired: 3 out]
        n268 = global read "GSP_SLIT_Global.vi" "Slit#"() -> (w561:i32)
        n269 = Number To Decimal String(number=w561) -> (decimal integer string=w560:string)  [unwired: 1 in]
        n270 = call <vilib>:"Write Characters To File.vi"("append to file? (new file:F)"=FALSE, "character string"=w560, "file path (dialog if empty)"=w554) -> ("new file path (Not A Path if cancelled)"=w558:path)  [unwired: 2 in]
        n271 = global write "GSP_SLIT_Global.vi" "Slit Rot State"(MotorStates."Moving" ("Rotation Mode")) -> ()
        n272 = Number To Decimal String(number=w556) -> (decimal integer string=w551:string)  [unwired: 1 in]
        n273 = Concatenate Strings("\r\n", w551) -> (w553:string)
        n274 = call <vilib>:"Write Characters To File.vi"("append to file? (new file:F)"=TRUE, "character string"=w553, "file path (dialog if empty)"=w558) -> ()  [unwired: 2 in, 1 out]
      }
      frame "SHUTDOWN" {
        n275 = Build Array(w588, w587) -> (w586:T4[])
        n276 = call "CalcSystemState.vi"("Motor States"=w586) -> ("system state"=w585:T4)
        n277 = case shown="\"Ready\", Default" w585 {
          tunnel: w592 -> [w597 w614 w619]
          tunnel: [w596 w614 w619] -> w591
          tunnel: w584 -> [w598 w613 w618]
          tunnel: w590 -> [_ w612 w617]
          tunnel: [w598 w611 w616] -> w589
          frame "Ready", Default {
            n278 = global read "GSP_SLIT_Global.vi" "Slit#"() -> (w595:i32)
            n279 = call "Build_Script.vi"("Commands"=cluster{"Command":string, "Parameters":string}[] [{"Command"="CLOSE_MASK", "Parameters"=""}, {"Command"="FINAL_SHUTDOWN", "Parameters"=""}]) -> ("script out"=w593:T2)  [unwired: 4 in]
            n280 = case shown="1, Default" w595 {
              selector: w595 -> [_ w603]
              tunnel: w597 -> [w601 w607]
              tunnel: [w600 w604] -> w596
              tunnel: w593 -> [w599 w602]
              frame 0 {
                n281 = Insert Into Array(array=w601, new element=w599) -> (w600:T1)  [unwired: 1 in]
              }
              frame 1, Default {
                n282 = call "SLIT_generate_script.vi"("Script Type"=enum16{"Home", "Change"}."Change", "Current Slit#"=w603, "Slit#"=0 ("Target")) -> ("script out"=w606:T2)
                n283 = Build Array(w606, w602) -> (w605:T2[])
                n284 = Insert Into Array(array=w607, new element=w605) -> (w604:T1)  [unwired: 1 in]
              }
            }
          }
          frame "Uninitialized" {
            n285 = Enqueue Element At Opposite End(queue=w612, element=cluster{"Command":string, "Parameters":string} {"Command"="FINAL_SHUTDOWN", "Parameters"=""}, error in (no error)=w613) -> (error out=w611:errorcluster)  [unwired: 1 in, 2 out]
          }
          frame "Error" {
            n286 = Enqueue Element At Opposite End(queue=w617, element=cluster{"Command":string, "Parameters":string} {"Command"="FINAL_SHUTDOWN", "Parameters"=""}, error in (no error)=w618) -> (error out=w616:errorcluster)  [unwired: 1 in, 2 out]
          }
        }
      }
      frame "FINAL_SHUTDOWN" {
        w623 = u8 2 ("Disabled")
        n287 = Release Queue(queue=w627, error in (no error)=w626) -> (error out=w620:errorcluster)  [unwired: 1 in, 2 out]
        n288 = global write "GSP_SLIT_Global.vi" "Slit Thread State"(ThreadStates."Uninitialized" ("Thread state")) -> ()
        n289 = property on="Slit Mask#" class="Ring (strict)"(error in=w620, "Disabled"=w623) -> (error out=w625:errorcluster)  [unwired: 1 in, 1 out]
        n290 = property on="Mask bump" class="Slide (strict)"(error in=w625, "Disabled"=w623) -> (error out=w624:errorcluster)  [unwired: 1 in, 1 out]
        n291 = property on="Hide Slit" class="Bool (strict)"(error in=w624, "Disabled"=w623) -> (error out=w622:errorcluster)  [unwired: 1 in, 1 out]
        n292 = stacked-sequence {
          tunnel: w622 -> [_]
          frame #0 {
            n293 = global write "GSP_SLIT_Global.vi" "Slit Online"(FALSE ("CS Online")) -> ()
          }
        }
      }
      frame "HOME" {
        w632 = MotorStates."Ready" ("Translation Mode")
        n294 = global read "GSP_SLIT_Global.vi" "Slit#"() -> (w631:i32)
        n295 = global write "GSP_SLIT_Global.vi" "Slit Trans State"(w632) -> ()
        n296 = global write "GSP_SLIT_Global.vi" "Slit Rot State"(w632) -> ()
        n297 = call "SLIT_generate_script.vi"("Script Type"=enum16{"Home", "Change"}."Home", "Current Slit#"=w631, "Slit#"=0) -> ("script out"=w633:T2)
        n298 = Insert Into Array(array=w637, new element=w633) -> (w636:T1)  [unwired: 1 in]
      }
      frame "HOME_START" {
        n299 = Unbundle By Name(w641) -> ("Trans Home Mem Address"=w640:i32, "Rot Home Mem Address"=w639:i32)
        n300 = Number To Decimal String(number=w639) -> (decimal integer string=w647:string)  [unwired: 1 in]
        n301 = Build Array(w647) -> (w646:string[])
        n302 = Number To Decimal String(number=w640) -> (decimal integer string=w645:string)  [unwired: 1 in]
        n303 = call "gsp_silvermax_commandreponse.vi"("error in (no error)"=w638, "Parameters (none)"=w646, "Motor #"=w653, "Command"=T5."LRP (156)") -> ("error out"=w652:errorcluster)  [unwired: 3 out]
        n304 = Build Array(w645) -> (w644:string[])
        n305 = call "gsp_silvermax_commandreponse.vi"("error in (no error)"=w652, "Parameters (none)"=w644, "Motor #"=w642, "Command"=T5."LRP (156)") -> ("error out"=w651:errorcluster)  [unwired: 3 out]
        n306 = case shown="No Error" w651 {
          selector: w651 -> [w655 w656]
          tunnel: [w655 w656] -> w650
          frame No Error {
            w654 = MotorStates."Moving" ("Translation Mode")
            n307 = global write "GSP_SLIT_Global.vi" "Slit Rot State"(w654) -> ()
            n308 = global write "GSP_SLIT_Global.vi" "Slit Trans State"(w654) -> ()
          }
          frame Error {
          }
        }
      }
      frame "ERROR" {
        n309 = local read "Last Error"() -> (w660:errorcluster)
        n310 = Unbundle By Name(w660) -> ("code"=w666:i32)
        n311 = Bundle By Name(cluster=T10 {"error in (no error)"={"status"=FALSE, "code"=0, "source"=""}, "Source"="", "Comment "=""} ("Log"), "error in (no error)"=w660, "Source"="Slit Manager") -> (w661:T10)
        n312 = call "GSP_Logger_Handler.vi"("Log"=w661, "Actions"=T9."Log") -> ()  [unwired: 5 in, 1 out]
        n313 = case shown="0, Default" w666 {
          tunnel: w660 -> [_ _ _]
          tunnel: [errorcluster {"status"=FALSE, "code"=0, "source"=""} ("Last Error") errorcluster {"status"=FALSE, "code"=0, "source"=""} ("Last Error") errorcluster {"status"=FALSE, "code"=0, "source"=""} ("Last Error")] -> w665
          tunnel: w658 -> [_ w675 w677]
          tunnel: [T1 [] ("Operations") w675 w677] -> w657
          frame 0, Default {
            w672 = MotorStates."Error" ("Rotation Mode")
            w670 = u8 2 ("Disabled")
            n314 = global write "GSP_SLIT_Global.vi" "Slit Thread State"(ThreadStates."Error" ("Thread state")) -> ()
            n315 = property on="Slit Mask#" class="Ring (strict)"("Disabled"=w670) -> ()  [unwired: 2 in, 2 out]
            n316 = property on="Hide Slit" class="Bool (strict)"("Disabled"=w670) -> ()  [unwired: 2 in, 2 out]
            n317 = property on="Mask bump" class="Slide (strict)"("Disabled"=w670) -> ()  [unwired: 2 in, 2 out]
            n318 = global write "GSP_SLIT_Global.vi" "Slit Rot State"(w672) -> ()
            n319 = global write "GSP_SLIT_Global.vi" "Slit Trans State"(w672) -> ()
          }
          frame 5003, 5006 {
          }
          frame 5013 {
          }
        }
        n320 = case shown="No Error" w665 {
          tunnel: w664 -> [_ w668]
          frame No Error {
          }
          frame Error {
            n321 = Enqueue Element At Opposite End(queue=w668, element=cluster{"Command":string, "Parameters":string} {"Command"="FINAL_SHUTDOWN", "Parameters"=""}) -> ()  [unwired: 2 in, 3 out]
          }
        }
      }
    }
    n322 = Equal?(x=w32, y="FINAL_SHUTDOWN") -> (x = y?=w33:bool)
    n323 = case shown="No Error" w41 {
      selector: w41 -> [_ w48]
      tunnel: w40 -> [_ w49]
      tunnel: w32 -> [_ w46]
      frame No Error {
      }
      frame Error {
        n324 = Bundle("element"="ERROR", "Command"=w46) -> (w45:cluster{"element":string, "Command":string})  [unwired: 1 in]
        n325 = Enqueue Element At Opposite End(queue=w49, element=w45) -> ()  [unwired: 2 in, 3 out]
        "Last Error" <- w48
      }
    }
  }
